vi "test Acyclic Loopback Selective Triggers.vi"(8 "error in":errorcluster, 11 "TestCase in":refnum<class "Octal Loopback.lvclass">) -> (0 "error out":errorcluster, 3 "TestCase out":refnum<class "Octal Loopback.lvclass">)   [LabVIEW 2020, in "Octal Loopback.lvclass"]
uses:
  Octal Loopback.lvclass
  C:/Program Files (x86)/National Instruments/LabVIEW 2020/vi.lib/NI/VeriStand Custom Device Testing Tools/VeriStandTestCase/VeriStandTestCase.lvclass
  <vilib>/numeric/Random Number (Range) U64.vi
  <vilib>/numeric/sub_Random U32.vi
  <vilib>/NI VeriStand/Execution/Workspace/NI VeriStand - Set Multiple Channel Values.vi
  <vilib>/addons/_JKI Toolkits/VI Tester/TestCase.llb/TestCase.lvclass
  <vilib>/NI VeriStand/Execution/Workspace/NI_VS Workspace ExecutionAPI.lvlib
  <vilib>/NI/VeriStand Custom Device Testing Tools/VeriStandTestUtilities/VeriStandTestUtilities.lvlib
  C:/Program Files (x86)/National Instruments/LabVIEW 2020/vi.lib/addons/_JKI Toolkits/VI Tester/TestCase.llb/TestCase.lvclass
  C:/Users/nitest/Desktop/Git 2020/niveristand-ballard-arinc429-custom-device/Source/Custom Device Support/Tests/System/Octal Loopback/Octal Loopback.lvclass
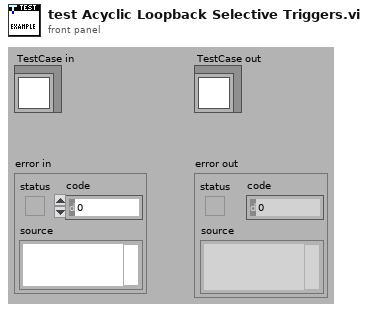
[diagram p1: front panel]
types:
  T1 = typedef "NI_VS Workspace ExecutionAPI.lvlib/WorkspaceAPI.ctl" = refnum<k24>
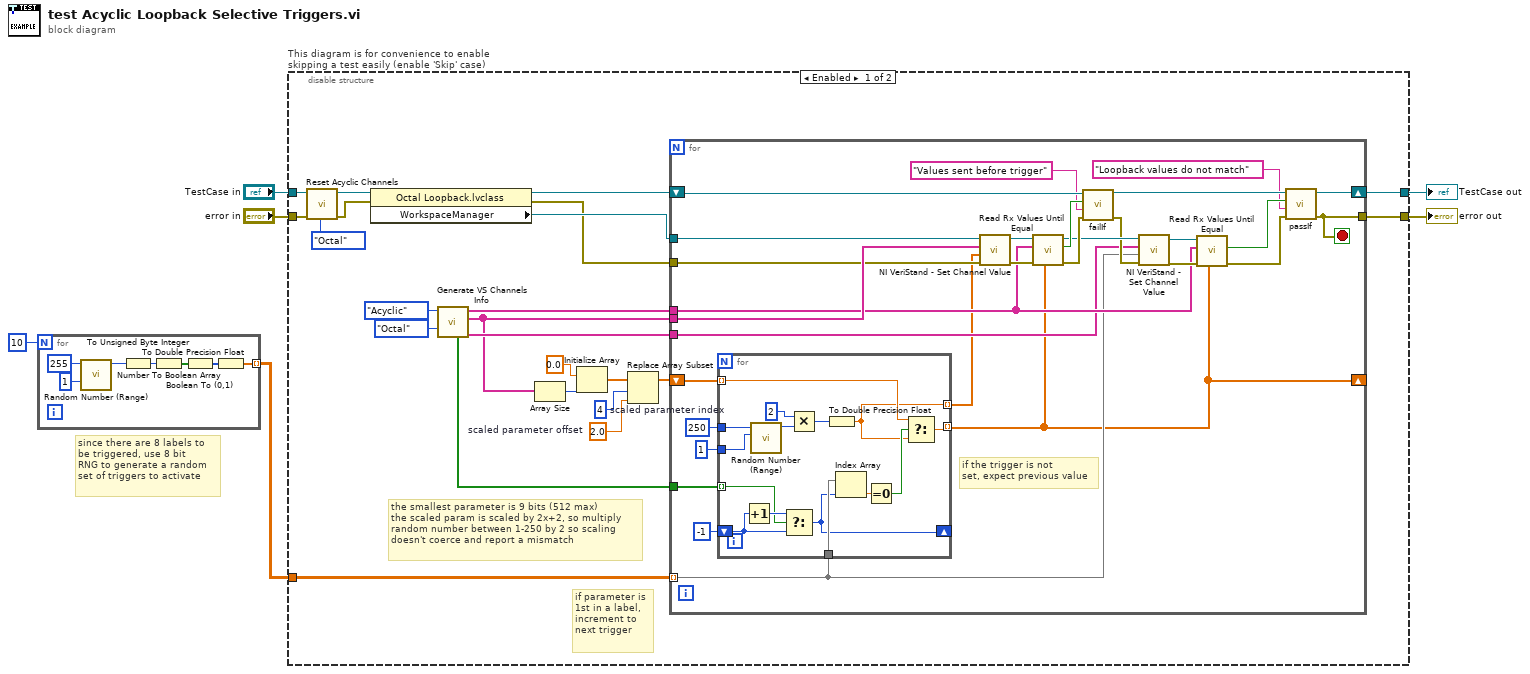
[diagram p0: block diagram]
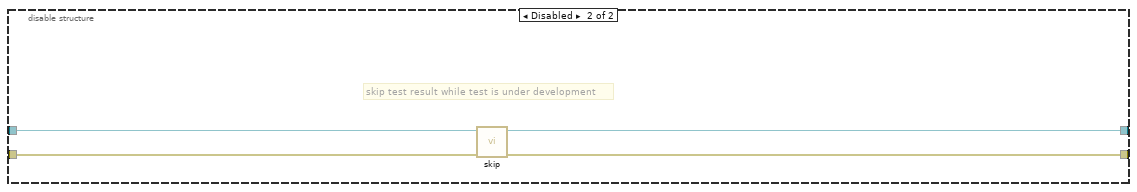
[diagram p2: hidden frame]
diagram:
  # "since there are 8 labels to\nbe triggered, use 8 bit \nRNG to generate a random\nset of triggers to activate"
  n1 = for {
    N: 10 -> [_]
    tunnel: [w7] -> w2 mode=indexing
    n2 = call-poly <vilib>:"Random Number (Range).vi"("lower bound (0)"=u64 1, "upper bound (100)"=u64 255) -> ("number"=w10:u64)  [unwired: 9 in]
    n3 = To Unsigned Byte Integer(number=w10) -> (unsigned 8bit integer=w9:u8)
    n4 = Number To Boolean Array(number=w9) -> (Boolean array=w13:bool[])
    n5 = Boolean To (0,1)(Boolean=w13) -> (0, 1=w8:i16[])
    n6 = To Double Precision Float(number=w8) -> (double precision float=w7:dbl[])
  }
  n7 = disable-structure "This diagram is for convenience to enable skipping a test easily (enable 'Skip' case)" shown="Enabled" {
    disable-tunnel: "TestCase in" -> [w16 w84]
    disable-tunnel: [w31 w82] -> w3
    disable-tunnel: [w30 w83] -> w5
    disable-tunnel: "error in" -> [w32 w81]
    disable-tunnel: w2 -> [w28 _]
    frame Enabled {
      w22 = 2.0  # scaled parameter offset
      w23 = 4  # scaled parameter index
      # "the smallest parameter is 9 bits (512 max)\nthe scaled param is scaled by 2x+2, so multiply \nrandom number between 1-250 by 2 so scaling\ndoesn't coerce and report a mismatch"
      # "if parameter is 1st in a label, increment to next trigger"
      n8 = call "Reset Acyclic Channels.vi"("error in (no error)"=w32, "Label Format (Decimal)"=enum16{"Decimal", "Octal"}."Octal", "reference in"=w16) -> ("error out"=w18:errorcluster, "reference out"=w17:refnum<class "Octal Loopback.lvclass">)  [unwired: 7 in]
      n9 = property class="Octal Loopback.lvclass"(reference=w17, error in=w18) -> (reference out=w33:refnum<class "Octal Loopback.lvclass">, error out=w34:errorcluster, "WorkspaceManager"=w35:T1)
      n10 = call "Generate VS Channels Info.vi"("Label Format (Decimal)"=enum16{"Decimal", "Octal"}."Octal", "Transfer Type"=enum16{"Acyclic", "Scheduled"}."Acyclic") -> ("Tx Trigger Channels Array"=w29:string[], "Tx Channels Array"=w21:string[], "Rx Channels Array"=w36:string[], "Is First Parameter? Array"=w20:bool[])  [unwired: 5 in, 1 out]
      n11 = Array Size(array=w21) -> (size(s)=w26:i32)
      n12 = Initialize Array(0.0 ("element"), w26) -> (w27:dbl[])
      n13 = Replace Array Subset(array=w27, new element=w22, index=w23) -> (w24:dbl[])
      n14 = for {
        tunnel: w36 -> [w51]
        tunnel: w35 -> [w63]
        tunnel: w34 -> [w56]
        tunnel: w21 -> [w62]
        shift-right: [w47] -> w31
        shift-left: w33 -> [w58]
        tunnel: [w46] -> w30
        tunnel: w29 -> [w43]
        tunnel: w28 -> [w42] mode=indexing
        shift-right: [w39] -> _
        shift-left: w24 -> [w40]
        tunnel: w20 -> [w37]
        stop <- w46 stop-if-true
        # "if the trigger is not\nset, expect previous value"
        n15 = for {
          tunnel: [w70] -> w39 mode=indexing
          tunnel: u64 250 ("upper bound (100)") -> [w79]
          tunnel: u64 1 ("upper bound (100)") -> [w78]
          tunnel: w42 -> [w75]
          shift-right: [w74] -> _
          shift-left: -1 -> [w72]
          tunnel: w40 -> [w68] mode=indexing
          tunnel: [w67] -> w38 mode=indexing
          tunnel: w37 -> [w66] mode=indexing
          n16 = Increment(x=w72) -> (x+1=w73:i32)
          n17 = call-poly <vilib>:"Random Number (Range).vi"("lower bound (0)"=w78, "upper bound (100)"=w79) -> ("number"=w80:u64)  [unwired: 9 in]
          n18 = Select(t=w73, s=w66, f=w72) -> (s? t:f=w74:i32)
          n19 = Multiply(x=u64 2, y=w80) -> (x*y=w77:u64)
          n20 = To Double Precision Float(number=w77) -> (double precision float=w67:dbl)
          n21 = Index Array(array=w75, index=w74) -> (element=w71:dbl)
          n22 = Equal To 0?(x=w71) -> (x = 0?=w69:bool)
          n23 = Select(t=w68, s=w69, f=w67) -> (s? t:f=w70:dbl)
        }
        n24 = call-poly <vilib>:"NI VeriStand - Set Channel Value.vi"("error in (no error)"=w56, "Values"=w38, "Channels"=w62, "WorkspaceManager in"=w63) -> ("error out"=w59:errorcluster, "WorkspaceManager out"=w61:T1)  [unwired: 6 in]
        n25 = call <vilib>:"Read Rx Values Until Equal.vi"("expected values"=w39, "error in"=w59, "Rx aliases"=w51, "workspace manager in"=w61) -> ("error out"=w60:errorcluster, "values equal expected"=w57:bool, "workspace manager out"=w55:T1)  [unwired: 5 in]
        n26 = call-dynamic "failIf.vi"("error in (no error)"=w60, "message (\"\")"="Values sent before trigger" ("message (\"\")"), "fail"=w57, "TestCase in"=w58) -> ("error out"=w54:errorcluster, "TestCase out"=w48:refnum<class "Octal Loopback.lvclass">)  [unwired: 6 in]
        n27 = call-poly <vilib>:"NI VeriStand - Set Channel Value.vi"("error in (no error)"=w54, "Values"=w42, "Channels"=w43, "WorkspaceManager in"=w55) -> ("error out"=w52:errorcluster, "WorkspaceManager out"=w53:T1)  [unwired: 6 in]
        n28 = call <vilib>:"Read Rx Values Until Equal.vi"("expected values"=w39, "error in"=w52, "Rx aliases"=w51, "workspace manager in"=w53) -> ("error out"=w49:errorcluster, "values equal expected"=w50:bool)  [unwired: 5 in, 1 out]
        n29 = call-dynamic "passIf.vi"("error in (no error)"=w49, "message (\"\")"="Loopback values do not match" ("message (\"\")"), "pass"=w50, "TestCase in"=w48) -> ("error out"=w46:errorcluster, "TestCase out"=w47:refnum<class "Octal Loopback.lvclass">)  [unwired: 6 in]
      }
    }
    frame Disabled {
      # "skip test result while test is under development"
      n30 = call <vilib>:"skip.vi"("error in (no error)"=w81, "TestCase in"=w84) -> ("error out"=w83:errorcluster, "TestCase out"=w82:refnum<class "Octal Loopback.lvclass">)  [unwired: 8 in]
    }
  }
  "error out" <- w5
  "TestCase out" <- w3
